vi "故障告警分析.vi"(8 "告警代码":u16, 9 "故障代码":u16, 10 "运行步序":u16, 11 "参数":string) -> (2 "报警内容":T1, 3 "简易报警状态":cluster{"故障状态":string, "报警状态":string})   [LabVIEW 2016, in "斯坦道CODMn新电路板.lvlib"]
panel:
  # "1、注射泵水样阀口堵塞；\n2、注射泵阀过载或丝杆无动作。"
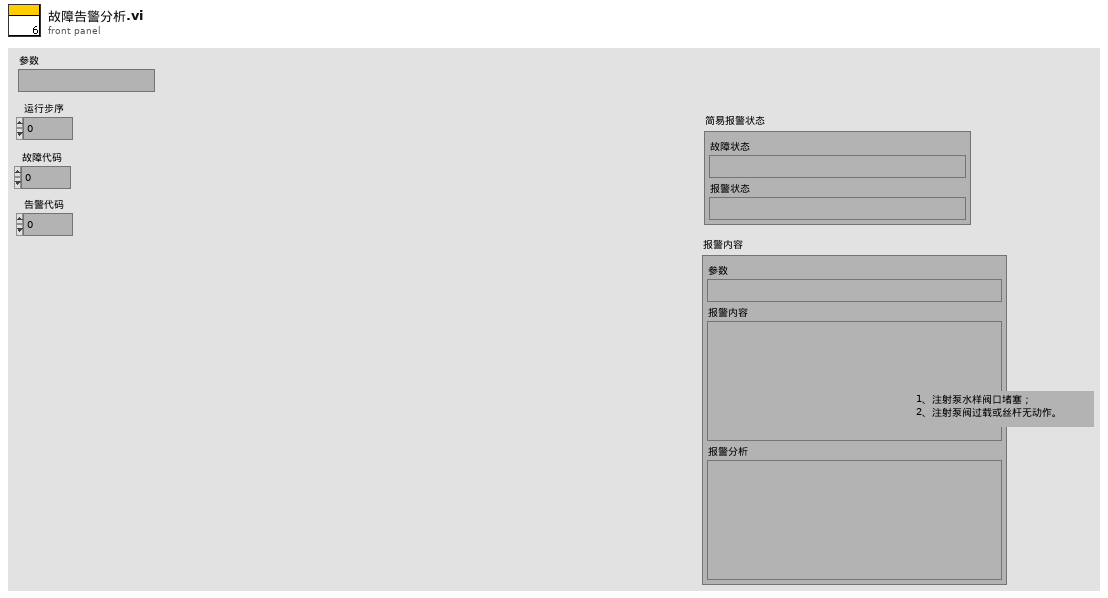
[diagram p1: front panel]
types:
  T1 = cluster{"参数":string, "报警内容":string, "报警分析":string}
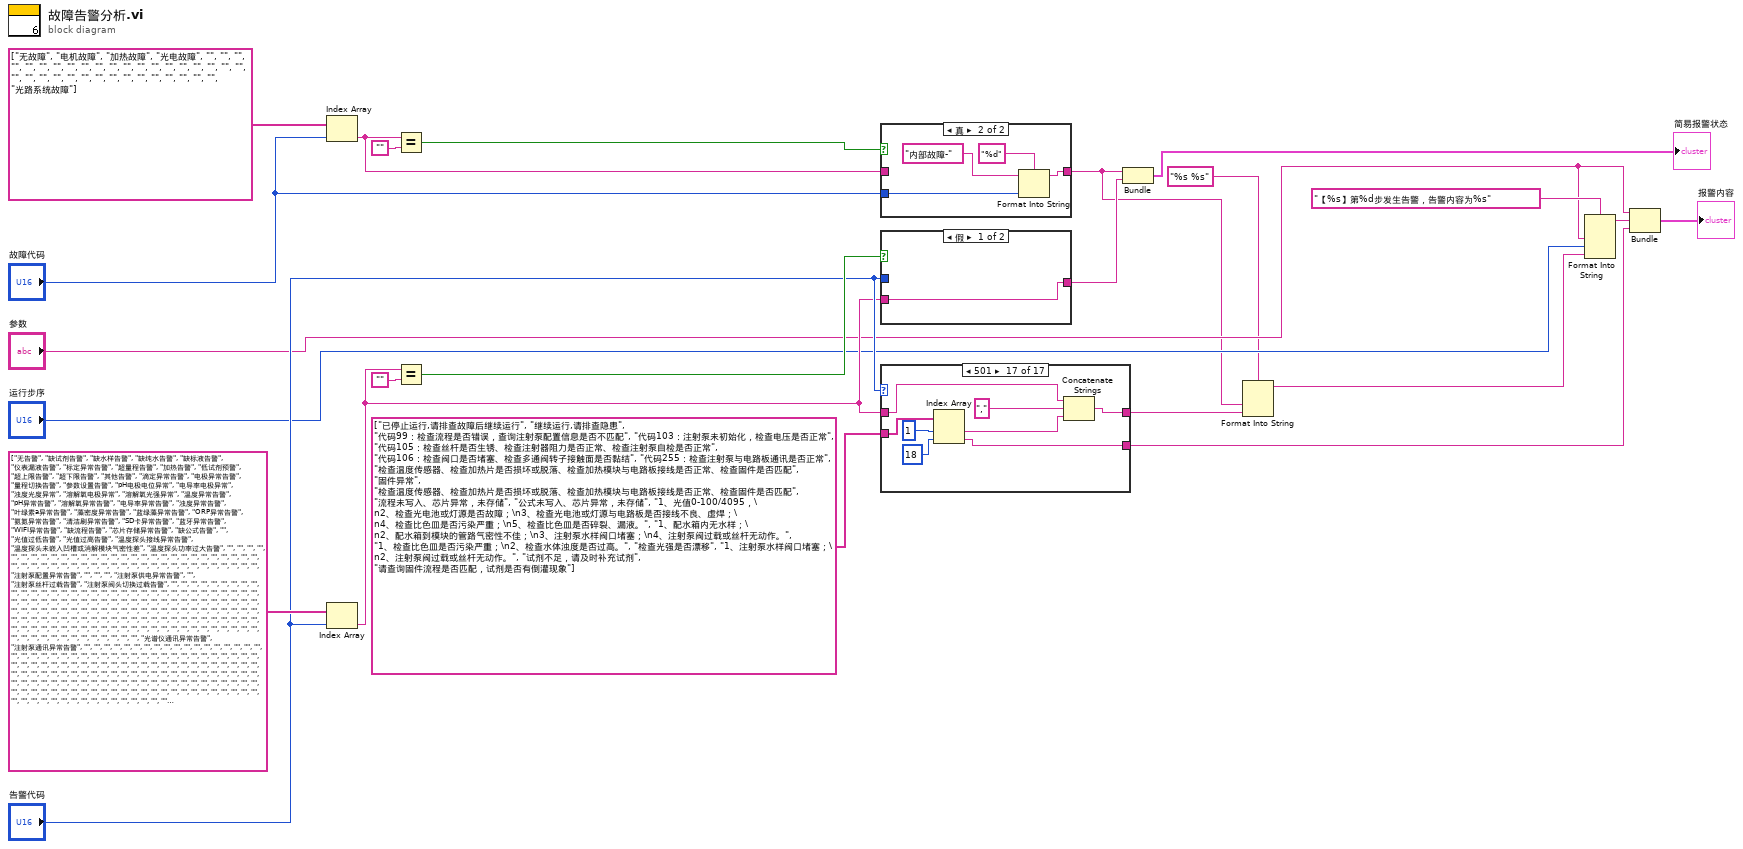
[diagram p0: block diagram]
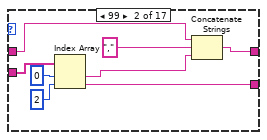
[diagram p3: hidden frame]
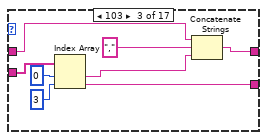
[diagram p4: hidden frame]
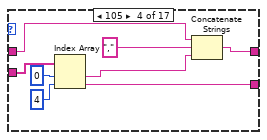
[diagram p5: hidden frame]
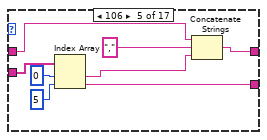
[diagram p6: hidden frame]
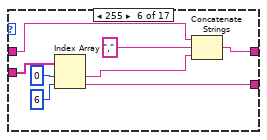
[diagram p7: hidden frame]
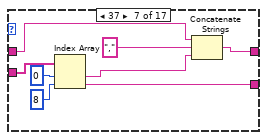
[diagram p8: hidden frame]
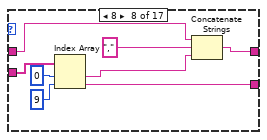
[diagram p9: hidden frame]
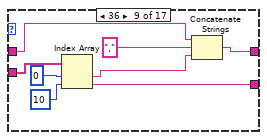
[diagram p10: hidden frame]
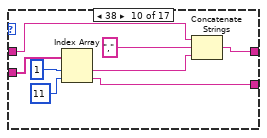
[diagram p11: hidden frame]
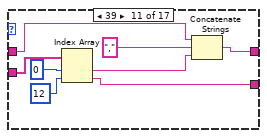
[diagram p12: hidden frame]
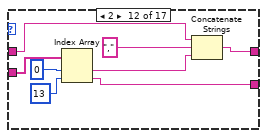
[diagram p13: hidden frame]
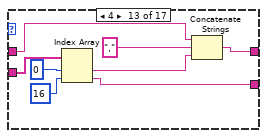
[diagram p14: hidden frame]
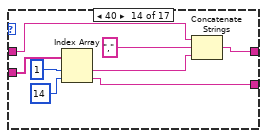
[diagram p15: hidden frame]
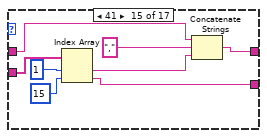
[diagram p16: hidden frame]
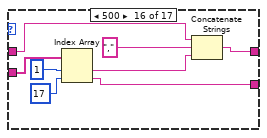
[diagram p17: hidden frame]
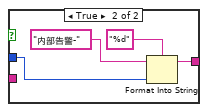
[diagram p18: hidden frame]
diagram:
  n1 = Index Array(array=string[] ["无故障", "电机故障", "加热故障", "光电故障", "", "", "", "", "", "", "", "", "", "", "", "", "", "", "", "", "", "", "", "", "", "", "", "", "", "", "", "", "", "", "", "", "", "", "", "光路系统故障"], index="故障代码") -> (element=w20:string)
  n2 = Index Array(array=string[] ["无告警", "缺试剂告警", "缺水样告警", "缺纯水告警", "缺标液告警", "仪表漏液告警", "标定异常告警", "超量程告警", "加热告警", "低试剂预警", "超上限告警", "超下限告警", "其他告警", "滴定异常告警", "电极异常告警", "量程切换告警", "参数设置告警", "pH电极电位异常", "电导率电极异常", "浊度光度异常", "溶解氧电极异常", "溶解氧光强异常", "温度异常告警", "pH异常告警", "溶解氧异常告警", "电导率异常告警", "浊度异常告警", "叶绿素a异常告警", "藻密度异常告警", "蓝绿藻异常告警", "ORP异常告警", "氨氮异常告警", "清洁刷异常告警", "SD卡异常告警", "蓝牙异常告警", "WIFI异常告警", "缺流程告警", "芯片存储异常告警", "缺公式告警", "", "光值过低告警", "光值过高告警", "温度探头接线异常告警", "温度探头未嵌入凹槽或消解模块气密性差", "温度探头功率过大告警", "", "", "", "", "", "", "", "", "", "", "", "", "", "", "", "", "", "", "", "", "", "", "", "", "", "", "", "", "", "", "", "", "", "", "", "", "", "", "", "", "", "", "", "", "", "", "", "", "", "", "", "", "", "", "注射泵配置异常告警", "", "", "", "注射泵供电异常告警", "", "注射泵丝杆过载告警", "注射泵阀头切换过载告警", "", "", "", "", "", "", "", "", "", "", "", "", "", "", "", "", "", "", "", "", "", "", "", "", "", "", "", "", "", "", "", "", "", "", "", "", "", "", "", "", "", "", "", "", "", "", "", "", "", "", "", "", "", "", "", "", "", "", "", "", "", "", "", "", "", "", "", "", "", "", "", "", "", "", "", "", "", "", "", "", "", "", "", "", "", "", "", "", "", "", "", "", "", "", "", "", "", "", "", "", "", "", "", "", "", "", "", "", "", "", "", "", "", "", "", "", "", "", "", "", "", "", "", "", "", "", "", "", "", "", "", "", "", "", "", "", "", "", "", "", "", "", "", "", "", "", "", "光谱仪通讯异常告警", "注射泵通讯异常告警", "", "", "", "", "", "", "", "", "", "", "", "", "", "", "", "", "", "", "", "", "", "", "", "", "", "", "", "", "", "", "", "", "", "", "", "", "", "", "", "", "", "", "", "", "", "", "", "", "", "", "", "", "", "", "", "", "", "", "", "", "", "", "", "", "", "", "", "", "", "", "", "", "", "", "", "", "", "", "", "", "", "", "", "", "", "", "", "", "", "", "", "", "", "", "", "", "", "", "", "", "", "", "", "", "", "", "", "", "", "", "", "", "", "", "", "", "", "", "", "", "", "", "", "", "", "", "", "", "", "", "", "", "", "", "", "", "", "", "", "", "", "", "", "", "", "", "", "", "", "", "", "", "", "", "", "", "", "", "", "", "", "", "", "", "", "", "", "", "", "", "", "", "", "", "", "", "", "", "", "", "", "", "", "", "", "", "", "", "", "", "", "", "", "", "", "", "", "", "", "", "", "", "", "", "", "", "", "", "", "", "", "", "", "", "", "", "", "", "", "", "", "", "", "", "", "", "", "", "", "", "", "", "", "", "", "", "", "", "", "", "", "", "", "", "试剂不足", "试剂余量检测异常"], index="告警代码") -> (element=w13:string)
  n3 = Equal?(x=w20, y="") -> (x = y?=w21:bool)
  n4 = Equal?(x=w13, y="") -> (x = y?=w16:bool)
  n5 = case shown="真" w21 {
    tunnel: [_ w25] -> w2
    tunnel: w20 -> [_ _]
    tunnel: "故障代码" -> [_ w24]
    frame False {
    }
    frame True {
      n6 = Format Into String(format string="%d" ("格式字符串"), initial string="内部故障-" ("工作状态"), w24) -> (resulting string=w25:string)  [unwired: 1 in, 1 out]
    }
  }
  n7 = case shown="假" w16 {
    tunnel: [w28 w30] -> w12
    tunnel: w13 -> [w28 _]
    tunnel: "告警代码" -> [_ w29]
    frame False {
    }
    frame True {
      n8 = Format Into String(format string="%d" ("格式字符串"), initial string="内部告警-" ("工作状态"), w29) -> (resulting string=w30:string)  [unwired: 1 in, 1 out]
    }
  }
  n9 = case shown="501" "告警代码" {
    tunnel: string[] ["已停止运行,请排查故障后继续运行", "继续运行,请排查隐患", "代码99：检查流程是否错误，查询注射泵配置信息是否不匹配", "代码103：注射泵未初始化，检查电压是否正常", "代码105：检查丝杆是否生锈、检查注射器阻力是否正常、检查注射泵自检是否正常", "代码106：检查阀口是否堵塞、检查多通阀转子接触面是否黏结", "代码255：检查注射泵与电路板通讯是否正常", "检查温度传感器、检查加热片是否损坏或脱落、检查加热模块与电路板接线是否正常、检查固件是否匹配", "固件异常", "检查温度传感器、检查加热片是否损坏或脱落、检查加热模块与电路板接线是否正常、检查固件是否匹配", "流程未写入、芯片异常，未存储", "公式未写入、芯片异常，未存储", "1、光值0-100/4095，\n2、检查光电池或灯源是否故障；\n3、检查光电池或灯源与电路板是否接线不良、虚焊；\n4、检查比色皿是否污染严重；\n5、检查比色皿是否碎裂、漏液。", "1、配水箱内无水样；\n2、配水箱到模块的管路气密性不佳；\n3、注射泵水样阀口堵塞；\n4、注射泵阀过载或丝杆无动作。", "1、检查比色皿是否污染严重；\n2、检查水体浊度是否过高。", "检查光强是否漂移", "1、注射泵水样阀口堵塞；\n2、注射泵阀过载或丝杆无动作。", "试剂不足，请及时补充试剂", "请查询固件流程是否匹配，试剂是否有倒灌现象"] -> [_ w41 w49 w57 w65 w73 w81 w89 w97 w105 w113 w121 w129 w137 w145 w153 w161]
    tunnel: [w33 w36 w44 w52 w60 w68 w76 w84 w92 w100 w108 w116 w124 w132 w140 w148 w156] -> w3
    tunnel: [_ w37 w45 w53 w61 w69 w77 w85 w93 w101 w109 w117 w125 w133 w141 w149 w157] -> w10
    tunnel: w13 -> [w33 w35 w43 w51 w59 w67 w75 w83 w91 w99 w107 w115 w123 w131 w139 w147 w155]
    frame 0, Default {
    }
    frame 99 {
      n10 = Index Array(array=w41, index #1=0 ("索引"), index #2=2 ("索引")) -> (element #1=w39:string, element #2=w37:string)
      n11 = Concatenate Strings(w35, "," ("字符串"), w39) -> (w36:string)
    }
    frame 103 {
      n12 = Index Array(array=w49, index #1=0 ("索引"), index #2=3 ("索引")) -> (element #1=w47:string, element #2=w45:string)
      n13 = Concatenate Strings(w43, "," ("字符串"), w47) -> (w44:string)
    }
    frame 105 {
      n14 = Index Array(array=w57, index #1=0 ("索引"), index #2=4 ("索引")) -> (element #1=w55:string, element #2=w53:string)
      n15 = Concatenate Strings(w51, "," ("字符串"), w55) -> (w52:string)
    }
    frame 106 {
      n16 = Index Array(array=w65, index #1=0 ("索引"), index #2=5 ("索引")) -> (element #1=w63:string, element #2=w61:string)
      n17 = Concatenate Strings(w59, "," ("字符串"), w63) -> (w60:string)
    }
    frame 255 {
      n18 = Index Array(array=w73, index #1=0 ("索引"), index #2=6 ("索引")) -> (element #1=w71:string, element #2=w69:string)
      n19 = Concatenate Strings(w67, "," ("字符串"), w71) -> (w68:string)
    }
    frame 37 {
      n20 = Index Array(array=w81, index #1=0 ("索引"), index #2=8 ("索引")) -> (element #1=w79:string, element #2=w77:string)
      n21 = Concatenate Strings(w75, "," ("字符串"), w79) -> (w76:string)
    }
    frame 8 {
      n22 = Index Array(array=w89, index #1=0 ("索引"), index #2=9 ("索引")) -> (element #1=w87:string, element #2=w85:string)
      n23 = Concatenate Strings(w83, "," ("字符串"), w87) -> (w84:string)
    }
    frame 36 {
      n24 = Index Array(array=w97, index #1=0 ("索引"), index #2=10 ("索引")) -> (element #1=w95:string, element #2=w93:string)
      n25 = Concatenate Strings(w91, "," ("字符串"), w95) -> (w92:string)
    }
    frame 38 {
      n26 = Index Array(array=w105, index #1=1 ("索引"), index #2=11 ("索引")) -> (element #1=w103:string, element #2=w101:string)
      n27 = Concatenate Strings(w99, "," ("字符串"), w103) -> (w100:string)
    }
    frame 39 {
      n28 = Index Array(array=w113, index #1=0 ("索引"), index #2=12 ("索引")) -> (element #1=w111:string, element #2=w109:string)
      n29 = Concatenate Strings(w107, "," ("字符串"), w111) -> (w108:string)
    }
    frame 2 {
      n30 = Index Array(array=w121, index #1=0 ("索引"), index #2=13 ("索引")) -> (element #1=w119:string, element #2=w117:string)
      n31 = Concatenate Strings(w115, "," ("字符串"), w119) -> (w116:string)
    }
    frame 4 {
      n32 = Index Array(array=w129, index #1=0 ("索引"), index #2=16 ("索引")) -> (element #1=w127:string, element #2=w125:string)
      n33 = Concatenate Strings(w123, "," ("字符串"), w127) -> (w124:string)
    }
    frame 40 {
      n34 = Index Array(array=w137, index #1=1 ("索引"), index #2=14 ("索引")) -> (element #1=w135:string, element #2=w133:string)
      n35 = Concatenate Strings(w131, "," ("字符串"), w135) -> (w132:string)
    }
    frame 41 {
      n36 = Index Array(array=w145, index #1=1 ("索引"), index #2=15 ("索引")) -> (element #1=w143:string, element #2=w141:string)
      n37 = Concatenate Strings(w139, "," ("字符串"), w143) -> (w140:string)
    }
    frame 500 {
      n38 = Index Array(array=w153, index #1=1 ("索引"), index #2=17 ("索引")) -> (element #1=w151:string, element #2=w149:string)
      n39 = Concatenate Strings(w147, "," ("字符串"), w151) -> (w148:string)
    }
    frame 501 {
      n40 = Index Array(array=w161, index #1=1 ("索引"), index #2=18 ("索引")) -> (element #1=w159:string, element #2=w157:string)
      n41 = Concatenate Strings(w155, "," ("字符串"), w159) -> (w156:string)
    }
  }
  n42 = Bundle(w2, w12) -> (→"简易报警状态":cluster{string, string})  [unwired: 1 in]
  n43 = Format Into String(format string="%s %s" ("格式字符串"), w2, w3) -> (resulting string=w4:string)  [unwired: 2 in, 1 out]
  n44 = Format Into String(format string="【%s】第%d步发生告警，告警内容为%s" ("格式字符串"), "参数", "运行步序", w4) -> (resulting string=w8:string)  [unwired: 2 in, 1 out]
  n45 = Bundle("参数"="参数", w8, w10) -> (→"报警内容":cluster{"参数":string, string, string})  [unwired: 1 in]
